vi "Audio Feedback Control.vi"(8 "error in (no error)":errorcluster, 10 "Audio Feedback":bool, 11 "Freq.":dbl) -> (0 "error out":errorcluster, 3 "task ID out":T1 format="%.0x")   [LabVIEW 2018, in "CollectionSupport.lvlib"]
uses:
  CollectionSupport.lvlib
  <vilib>/sound2/lvsound2.llb/Sound Output Task ID.ctl
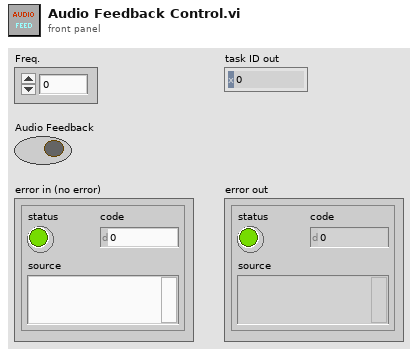
[diagram p1: front panel]
types:
  T1 = typedef "Sound Output Task ID.ctl" = u32
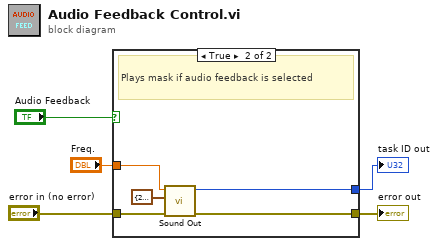
[diagram p0: block diagram]
diagram:
  n1 = case shown="True" "Audio Feedback" {
    tunnel: [w6 w11] -> w4
    tunnel: "Freq." -> [_ w10]
    tunnel: "error in (no error)" -> [w6 w8]
    tunnel: [_ w7] -> w5
    frame False {
    }
    frame True {
      # "Plays mask if audio feedback is selected"
      n2 = call "Sound Out.vi"("error in (no error)"=w8, "sampling info"=cluster{"Fs":dbl, "#s":dbl} {"Fs"=22050.0, "#s"=220500.0}, "Detected Frequency (Hz)"=w10) -> ("error out"=w11:errorcluster, "task ID out"=w7:T1)  [unwired: 7 in]
    }
  }
  "task ID out" <- w5
  "error out" <- w4
